vi "Understanding Arrays.vi"() -> ()   [LabVIEW 2026]
panel:
  out "Element Indicator":dbl
  in  "index":i32
  out "size(s)":i32
  out "Array 6":dbl[](array[slide]) scale=0.0..10.0
  in  "Array 5":dbl[](array[numeric])
  out "Array 2":dbl[](array[slide]) scale=0.0..10.0
  in  "Array":dbl[](array[numeric])
  in  "Array 3":bool[](array[boolean])
  out "Array 4":bool[](array[boolean])
  # "Understanding Arrays"
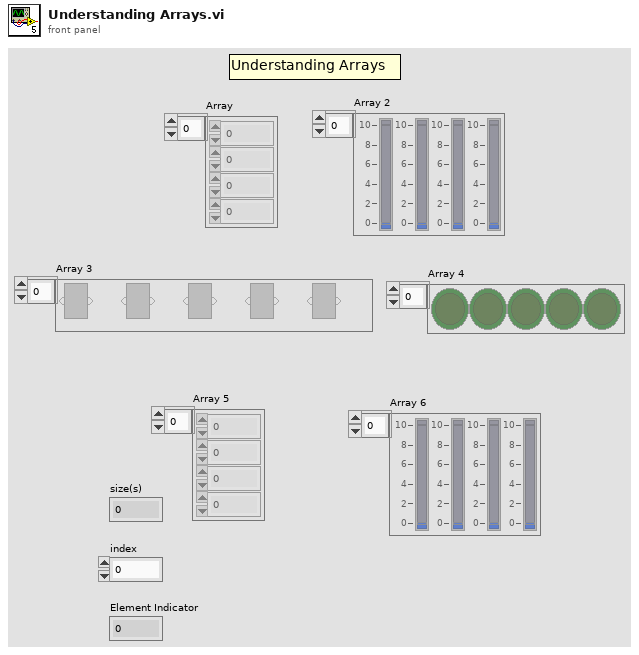
[diagram p1: front panel]
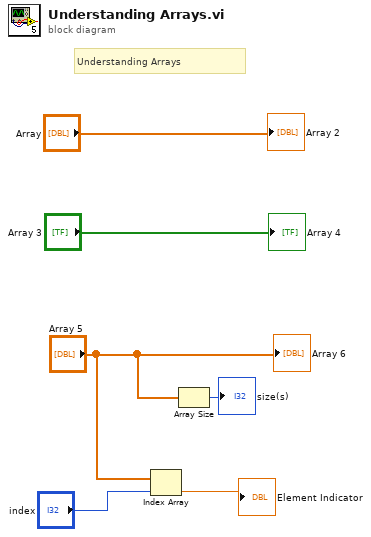
[diagram p0: block diagram]
diagram:
  # "Understanding Arrays"
  n1 = Index Array(array="Array 5", index="index") -> (element=→"Element Indicator":dbl)
  n2 = Array Size(array="Array 5") -> (size(s)=→"size(s)":i32)
  "Array 4" <- "Array 3"
  "Array 2" <- "Array"
  "Array 6" <- "Array 5"
